vi "GetDict.vi"(8 "error in (no error)":errorcluster caption="Fehler (Eingang, kein Fehler)", 11 "Dictionary (Eingang)":refnum<class "Dictionary.lvclass">) -> (0 "error out":errorcluster caption="Fehler (Ausgang)", 2 "Dict":variant, 3 "Dictionary (Ausgang)":refnum<class "Dictionary.lvclass">)   [LabVIEW 2013, in "Dictionary.lvclass"]
uses:
  Dictionary.lvclass
  Dictionary.lvclass/Dictionary.ctl
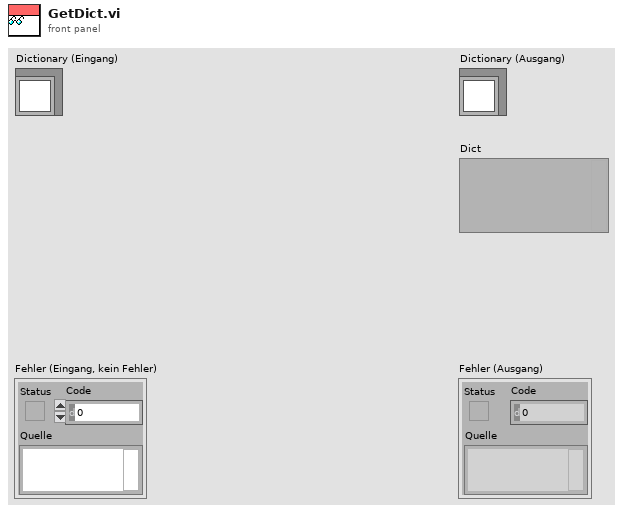
[diagram p1: front panel]
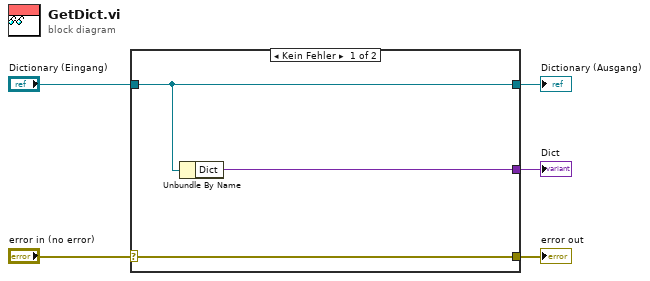
[diagram p0: block diagram]
diagram:
  n1 = case shown="Kein Fehler" "error in (no error)" {
    selector: "error in (no error)" -> [w8 w9]
    tunnel: [w8 w9] -> w4
    tunnel: [w7 w10] -> w2
    tunnel: "Dictionary (Eingang)" -> [w7 w10]
    tunnel: [w6 _] -> w1
    frame No Error {
      n2 = Unbundle By Name(w7) -> ("Dict"=w6:variant)
    }
    frame Error {
    }
  }
  "error out" <- w4
  "Dictionary (Ausgang)" <- w2
  "Dict" <- w1
